vi "New.vi"(6 "Timeout ms (25000)":i32=25000, 8 "Error In":errorcluster, 11 "Port (61557)":u16=61557) -> (0 "Error Out":errorcluster, 3 "UDP Ref.":refnum<class "UDP.lvclass">)   [LabVIEW 2020, in "RemoteVariables.lvlib" / "UDP.lvclass"]
uses:
  UDP.lvclass
  UDP.lvclass/UDP.ctl
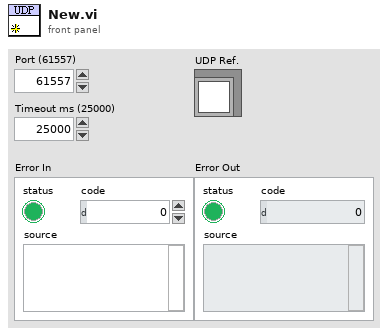
[diagram p1: front panel]
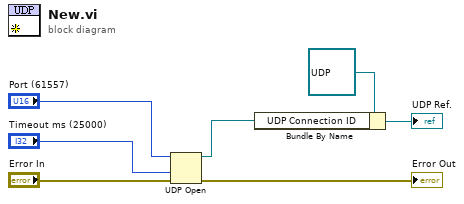
[diagram p0: block diagram]
diagram:
  n1 = UDP Open(8:"Error In", 9:"Timeout ms (25000)", 11:"Port (61557)") -> (port=w3:refnum<k16>, 0:→"Error Out":errorcluster)  [unwired: 2 in, 1 out]
  n2 = Bundle By Name(cluster=refnum<class "UDP.lvclass"> refnum ("RemoteVariables.lvlib:UDP.lvclass"), "UDP Connection ID"=w3) -> (→"UDP Ref.":refnum<class "UDP.lvclass">)
